vi "Read Limit(Boolean Array).vi"(7 "Test":string, 8 "error in (no error)":errorcluster) -> (0 "error out":errorcluster, 2 "a":bool[](array[boolean]), 3 "b":bool[](array[boolean]))   [LabVIEW 2019, in "Unit Test Engine Tools.lvlib"]
uses:
  Unit Test Engine Tools.lvlib
  LVUT Global 1.vi
  <vilib>/Utility/file.llb/Read Delimited Spreadsheet (string).vi
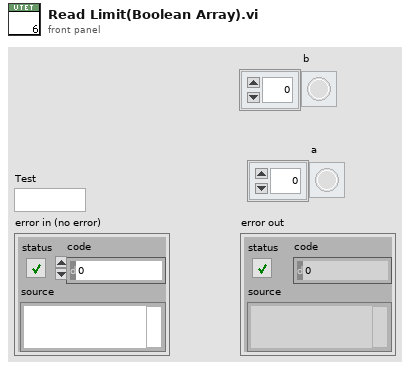
[diagram p1: front panel]
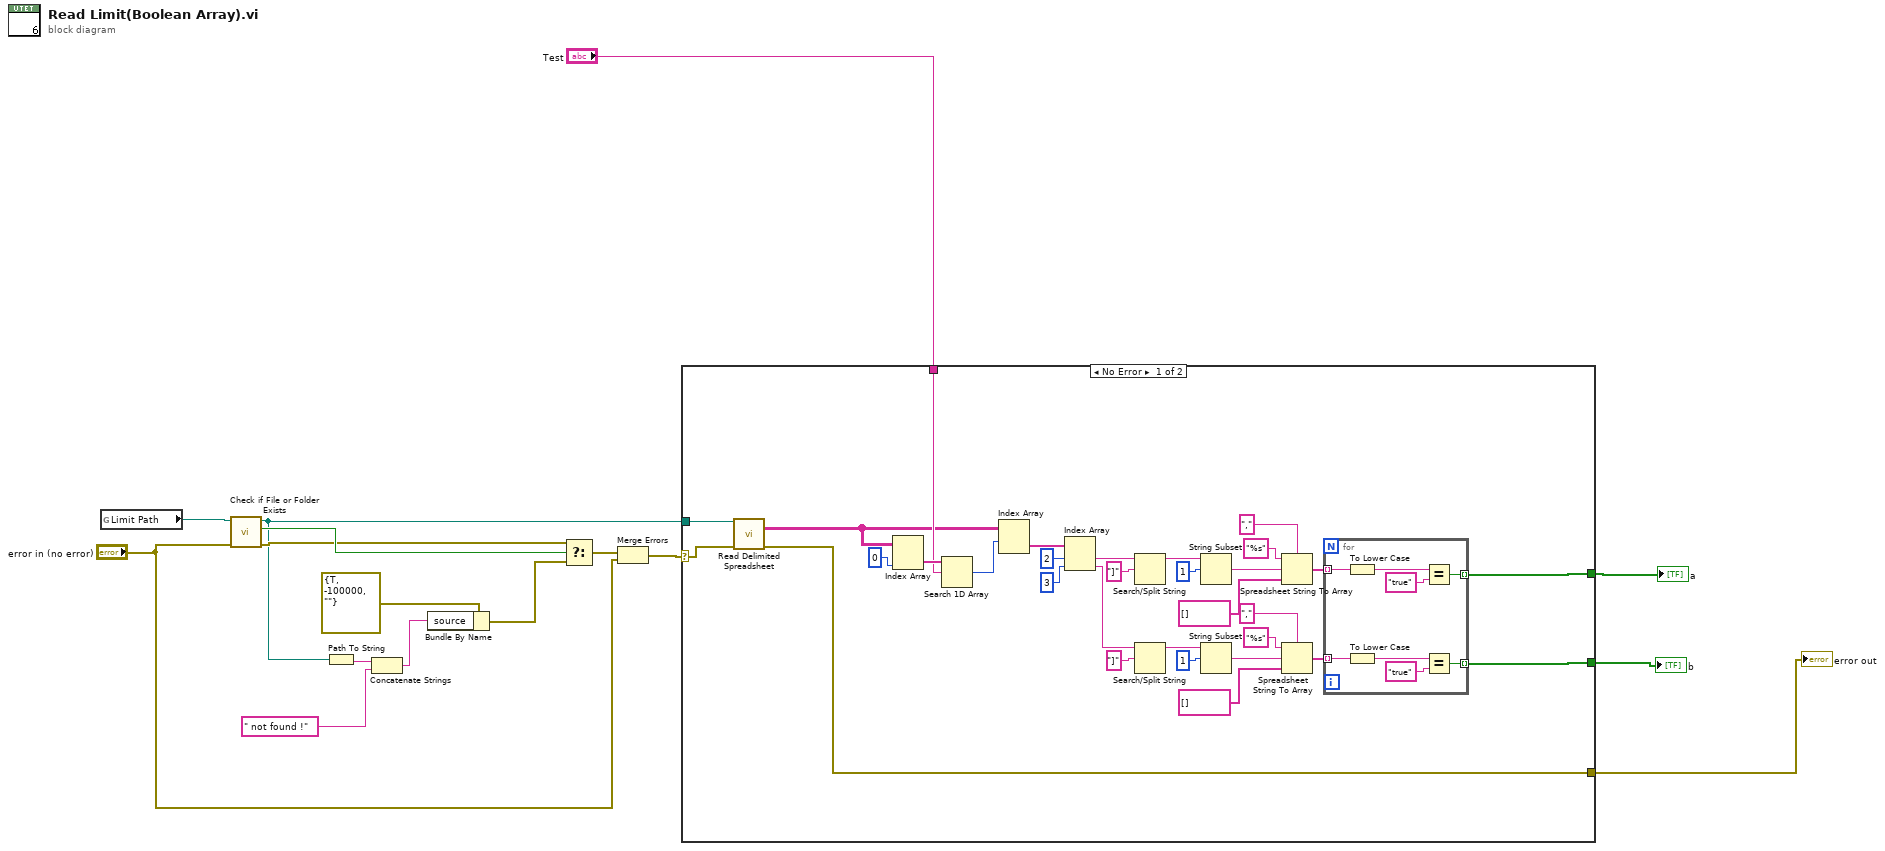
[diagram p0: block diagram]
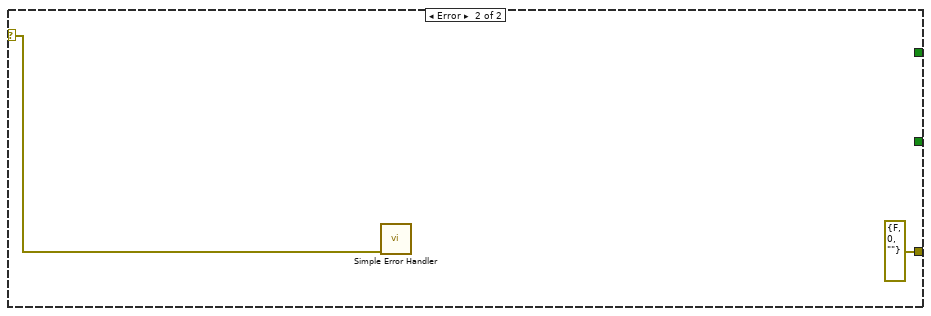
[diagram p2: hidden frame]
diagram:
  n1 = global read "LVUT Global 1.vi" "Limit Path"() -> (w13:path)
  n2 = call <vilib>:"Check if File or Folder Exists.vi"("error in (no error)"="error in (no error)", "path"=w13) -> ("error out"=w11:errorcluster, "file or folder exists?"=w12:bool, "dup path"=w6:path)  [unwired: 7 in]
  n3 = Path To String(path=w6) -> (string=w15:string)
  n4 = Concatenate Strings(w15, " not found !" ("string")) -> (w8:string)
  n5 = Bundle By Name(cluster=errorcluster {"status"=TRUE, "code"=-100000, "source"=""} ("f"), "source"=w8) -> (w9:errorcluster)
  n6 = Select(t=w11, s=w12, f=w9) -> (s? t:f=w7:errorcluster)
  n7 = Merge Errors(w7, "error in (no error)") -> (w4:errorcluster)
  n8 = case shown="No Error" w4 {
    selector: w4 -> [w18 w57]
    tunnel: "Test" -> [w45 _]
    tunnel: [w22 _] -> w1
    tunnel: [w20 _] -> w2
    tunnel: w6 -> [w19 _]
    tunnel: [w17 errorcluster {"status"=FALSE, "code"=0, "source"=""} ("error out")] -> w3
    frame No Error {
      n9 = call-poly <vilib>:"Read Delimited Spreadsheet.vi"("file path (dialog if empty)"=w19, "error in (no error)"=w18) -> ("all rows"=w44:string[][], "error out"=w17:errorcluster)  [unwired: 8 in, 4 out]
      n10 = Index Array(array=w44, index (col)=0 ("disabled index (col)")) -> (element=w46:string[])  [unwired: 1 in]
      n11 = Search 1D Array(1D array=w46, element=w45) -> (index of element=w43:i32)  [unwired: 1 in]
      n12 = Index Array(array=w44, index (row)=w43) -> (element=w42:string[])  [unwired: 1 in]
      n13 = Index Array(array=w42, index #1=2 ("index"), index #2=3 ("index")) -> (element #1=w26:string, element #2=w25:string)
      n14 = Search/Split String(string=w26, search string/char (-)="]" ("regular expression")) -> (substring before match=w38:string)  [unwired: 1 in, 2 out]
      n15 = Search/Split String(string=w25, search string/char (-)="]" ("regular expression")) -> (substring before match=w28:string)  [unwired: 1 in, 2 out]
      n16 = String Subset(string=w38, offset (0)=1) -> (substring=w39:string)  [unwired: 1 in]
      n17 = String Subset(string=w28, offset (0)=1) -> (substring=w27:string)  [unwired: 1 in]
      n18 = Spreadsheet String To Array(delimiter (Tab)=",", format string="%s", spreadsheet string=w39, array type (2D Dbl)=string[] []) -> (array=w23:string[])
      n19 = Spreadsheet String To Array(delimiter (Tab)=",", format string="%s", spreadsheet string=w27, array type (2D Dbl)=string[] []) -> (array=w21:string[])
      n20 = for {
        tunnel: w23 -> [w53] mode=indexing
        tunnel: [w52] -> w22 mode=indexing
        tunnel: w21 -> [w49] mode=indexing
        tunnel: [w48] -> w20 mode=indexing
        n21 = To Lower Case(string=w53) -> (all lower case string=w55:string)
        n22 = To Lower Case(string=w49) -> (all lower case string=w50:string)
        n23 = Equal?(x=w55, y="true") -> (x = y?=w52:bool)
        n24 = Equal?(x=w50, y="true") -> (x = y?=w48:bool)
      }
    }
    frame Error {
      n25 = call <vilib>:"Simple Error Handler.vi"("error in (no error)"=w57) -> ()  [unwired: 4 in, 5 out]
    }
  }
  "error out" <- w3
  "b" <- w2
  "a" <- w1
